vi "Cal7-GetCalNumbers.vi"(9 "CalString":string, 10 "StringName":string, 11 "EarlierPoints":bool) -> (1 "Array3":dbl[](array[numeric]), 2 "Array0":dbl[](array[numeric]), 3 "Array2":dbl[](array[numeric]), 4 "Array4":dbl[](array[numeric]), 5 "Array1":dbl[](array[numeric]), 6 "Array5":bool[](array[boolean]))   [LabVIEW 2016]
uses:
  Anemometry Sub Vis/Globals/Calib_global.vi
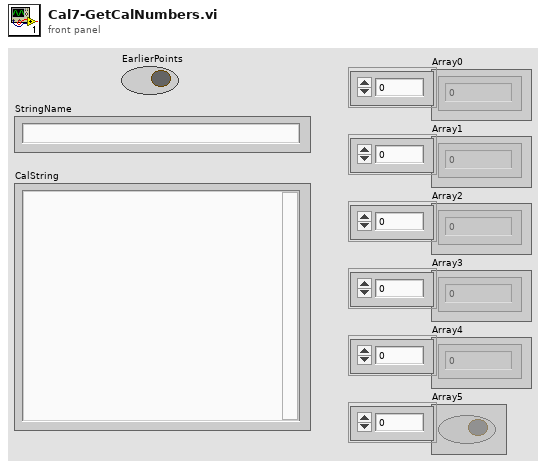
[diagram p1: front panel]
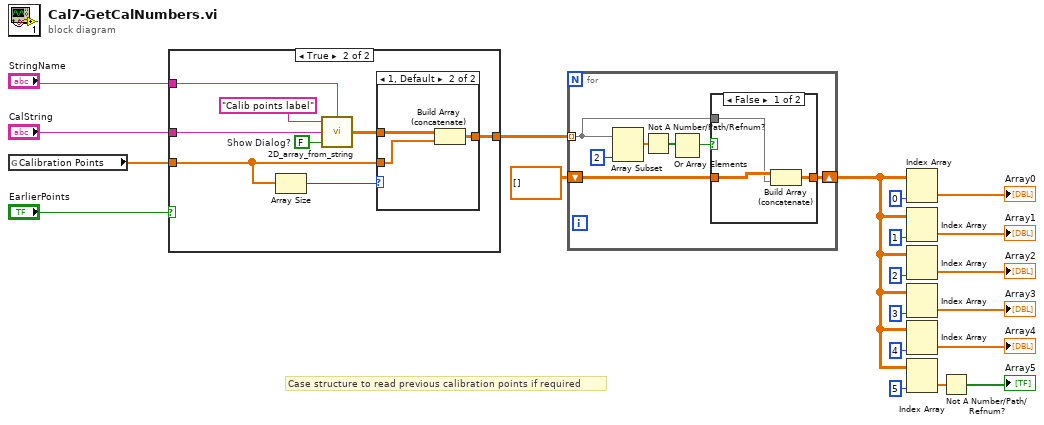
[diagram p0: block diagram]
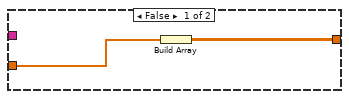
[diagram p3: hidden frame]
diagram:
  # "Case structure to read previous calibration points if required"
  n1 = global read "Calib_global.vi" "Calibration Points"() -> (w16:dbl[])
  n2 = case shown="True" "EarlierPoints" {
    tunnel: "CalString" -> [_ w29]
    tunnel: [w21 w26] -> w17
    tunnel: w16 -> [w22 w25]
    tunnel: "StringName" -> [_ w23]
    frame False {
      n3 = Build Array(w22) -> (w21:dbl[][])
    }
    frame True {
      w28 = FALSE  # Show Dialog?
      n4 = Array Size(array=w25) -> (size(s)=w24:i32)
      n5 = call "2D_array_from_string.vi"("String Name"=w23, "Show Dialog?"=w28, "Input string"=w29, "Array title"="Calib points label") -> ("2D data array"=w27:dbl[][])
      n6 = case shown="1, Default" w24 {
        tunnel: w27 -> [w31 w34]
        tunnel: [w31 w33] -> w26
        tunnel: w25 -> [_ w32]
        frame 0 {
        }
        frame 1, Default {
          n7 = Build Array (concatenate)(w34, w32) -> (w33:dbl[][])
        }
      }
    }
  }
  n8 = for {
    tunnel: w17 -> [w35] mode=indexing
    shift-right: [w36] -> w19
    shift-left: dbl[][] [] -> [w37]
    n9 = Array Subset(array=w35, length=2) -> (w40:dbl[])  [unwired: 1 in]
    n10 = Not A Number/Path/Refnum?(number/path/refnum=w40) -> (NaN/Path/Refnum?=w39:bool[])
    n11 = Or Array Elements(Boolean array=w39) -> (logical OR=w38:bool)
    n12 = case shown="False" w38 {
      tunnel: w37 -> [w44 w45]
      tunnel: w35 -> [w43 _]
      tunnel: [w42 w45] -> w36
      frame False {
        n13 = Build Array (concatenate)(w44, w43) -> (w42:dbl[][])
      }
      frame True {
      }
    }
  }
  n14 = Index Array(array=w19, index (col)=0) -> (element=→"Array0":dbl[])  [unwired: 1 in]
  n15 = Index Array(array=w19, index (col)=1) -> (element=→"Array1":dbl[])  [unwired: 1 in]
  n16 = Index Array(array=w19, index (col)=2) -> (element=→"Array2":dbl[])  [unwired: 1 in]
  n17 = Index Array(array=w19, index (col)=3) -> (element=→"Array3":dbl[])  [unwired: 1 in]
  n18 = Index Array(array=w19, index (col)=4) -> (element=→"Array4":dbl[])  [unwired: 1 in]
  n19 = Index Array(array=w19, index (col)=5) -> (element=w12:dbl[])  [unwired: 1 in]
  n20 = Not A Number/Path/Refnum?(number/path/refnum=w12) -> (NaN/Path/Refnum?=→"Array5":bool[])
